vi "Get Textbox Reference.vi"(8 "error in (no error)":errorcluster, 10 "VI reference (calling)":refnum<vi>, 11 "Dialog in":refnum<class "Dialog.lvclass">) -> (0 "error out":errorcluster, 2 "VI reference (dup)":refnum<vi>, 3 "Dialog out":refnum<class "Dialog.lvclass">)   [LabVIEW 2012, in "Dialog.lvlib" / "Dialog.lvclass"]
uses:
  Dialog.lvclass
  Dialog.lvclass/Dialog.ctl
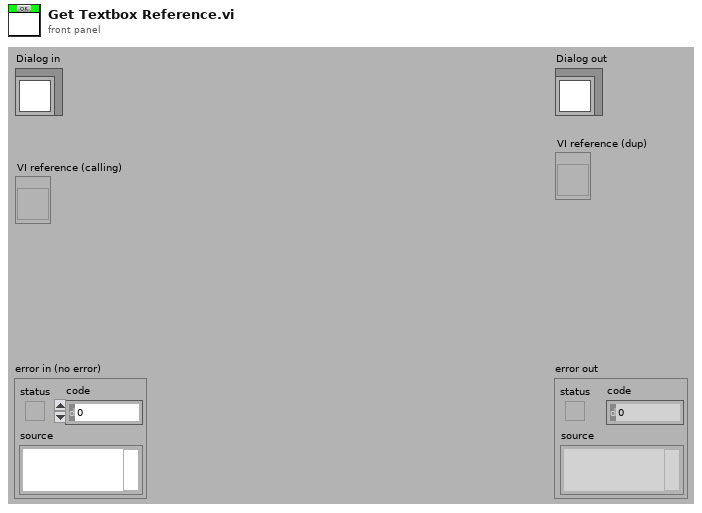
[diagram p1: front panel]
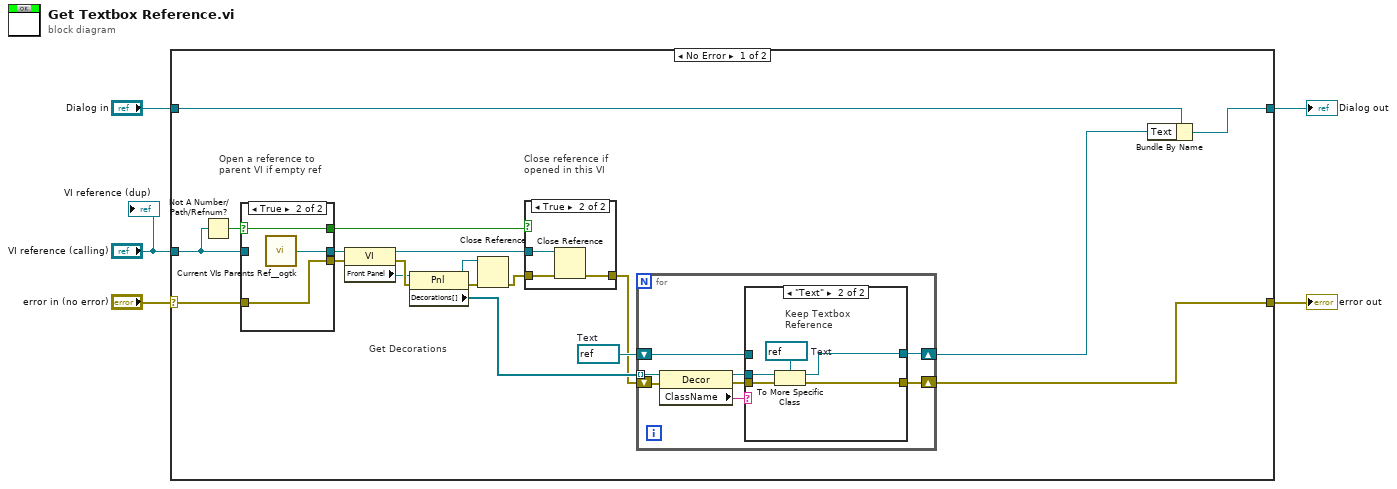
[diagram p0: block diagram]
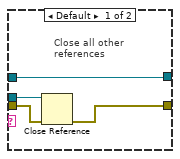
[diagram p2: hidden frame]
diagram:
  n1 = case shown="No Error" "error in (no error)" {
    selector: "error in (no error)" -> [w17 w53]
    tunnel: [w7 w53] -> w4
    tunnel: [w21 w52] -> w2
    tunnel: "Dialog in" -> [w22 w52]
    tunnel: "VI reference (calling)" -> [w18 _]
    frame No Error {
      w9 = refnum<vi> refnum  # Text
      # "Get Decorations"
      # "Close reference if\nopened in this VI"
      # "Open a reference to\nparent VI if empty ref"
      n2 = Not A Number/Path/Refnum?(number/path/refnum=w18) -> (NaN/Path/Refnum?=w20:bool)
      n3 = case shown="True" w20 {
        selector: w20 -> [w47 w51]
        tunnel: [w47 w51] -> w15
        tunnel: [w48 w50] -> w19
        tunnel: w18 -> [w48 _]
        tunnel: w17 -> [w46 w49]
        tunnel: [w46 w49] -> w16
        frame False {
        }
        frame True {
          n4 = call <userlib>:"Current VIs Parents Ref__ogtk.vi"() -> ("Calling VI's Reference"=w50:refnum<vi>)  [unwired: 2 out]
        }
      }
      n5 = property on="Property Node" class="VI"(reference=w19, error in=w16) -> (reference out=w14:refnum<vi>, error out=w24:errorcluster, "Front Panel"=w23:refnum<vi>)
      n6 = property on="Property Node" class="Pnl"(reference=w23, error in=w24) -> (reference out=w12:refnum<vi>, error out=w13:errorcluster, "Decorations[]"=w10:refnum<vi>[])
      n7 = Close Reference(reference=w12, error in (no error)=w13) -> (error out=w11:errorcluster)
      n8 = case shown="True" w15 {
        tunnel: w14 -> [_ w45]
        tunnel: [w42 w44] -> w8
        tunnel: w11 -> [w42 w43]
        frame False {
        }
        frame True {
          n9 = Close Reference(reference=w45, error in (no error)=w43) -> (error out=w44:errorcluster)
        }
      }
      n10 = for {
        tunnel: w10 -> [w25] mode=indexing
        shift-right: [w30] -> w6
        shift-left: w9 -> [w29]
        shift-right: [w27] -> w7
        shift-left: w8 -> [w26]
        n11 = property class="Decor"(reference=w25, error in=w26) -> (reference out=w32:refnum<vi>, error out=w28:errorcluster, "ClassName"=w31:string)
        n12 = case shown="\"Text\"" w31 {
          tunnel: w32 -> [w33 w40]
          tunnel: [w36 w39] -> w30
          tunnel: w29 -> [w36 _]
          tunnel: w28 -> [w35 w38]
          tunnel: [w34 w37] -> w27
          frame Default {
            # "Close all other\nreferences"
            n13 = Close Reference(reference=w33, error in (no error)=w35) -> (error out=w34:errorcluster)
          }
          frame "Text" {
            w41 = refnum<vi> refnum  # Text
            # "Keep Textbox\nReference"
            n14 = To More Specific Class(target class=w41, reference=w40, error in=w38) -> (specific class reference=w39:refnum<vi>, error out=w37:errorcluster)
          }
        }
      }
      n15 = Bundle By Name(cluster=w22, "Text"=w6) -> (w21:refnum<class "Dialog.lvclass">)
    }
    frame Error {
    }
  }
  "error out" <- w4
  "Dialog out" <- w2
  "VI reference (dup)" <- "VI reference (calling)"
